vi "FP_pattern.vi"() -> ()   [LabVIEW 2014]
uses:
  Between.vi
panel:
  out "output cluster":cluster{i16, "Bottom":i16}
  in  "stop":bool caption="(F4)"
  in  "Picture":picture
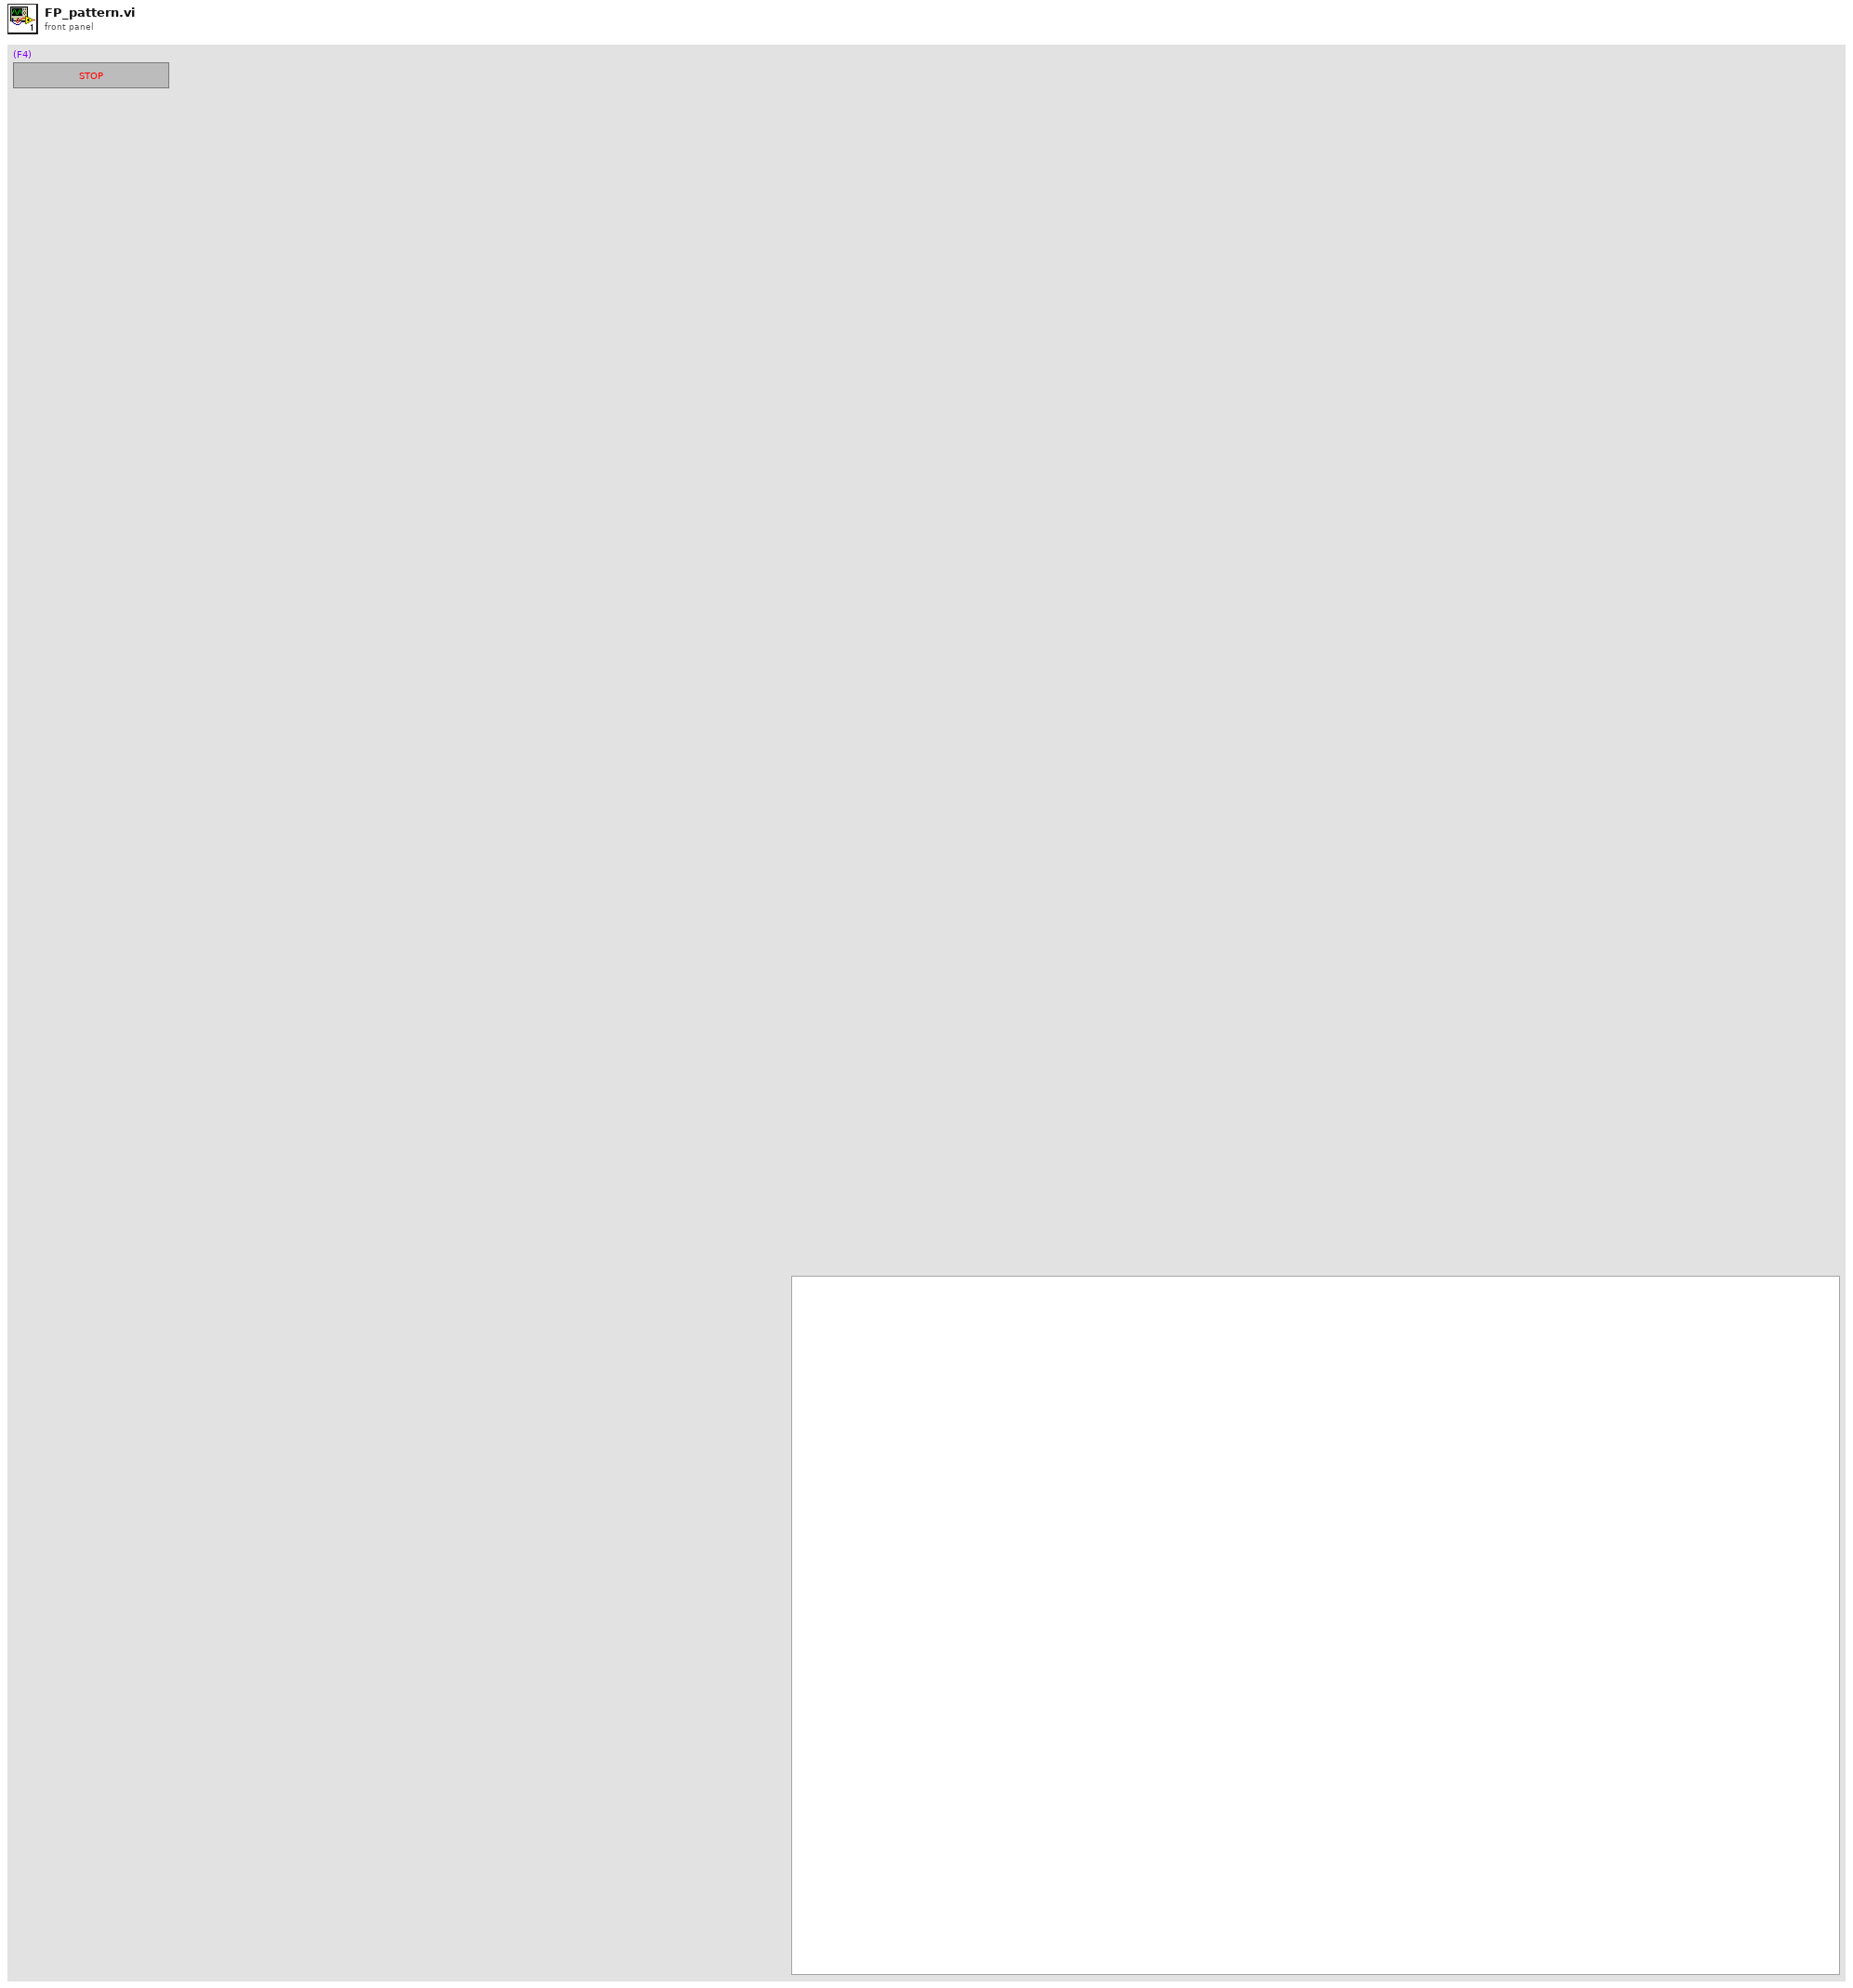
[diagram p1: front panel]
types:
  T1 = typedef "LVAllMonitorsDisplayTypeDef.ctl" = cluster{"Bounds":cluster{"Left":i16, "Top":i16, "Right":i16, "Bottom":i16}, "Depth":i16}[]
  T2 = cluster{"Bounds":cluster{"Left":i16, "Top":i16, "Right":i16, "Bottom":i16}, "Depth":i16}
  T3 = cluster{"Left":i16, "Top":i16, "Right":i16, "Bottom":i16}
  T4 = cluster{"Width":u16, "Style":enum32{"Solid", "Dash", "Dot", "DashDot", "DashDotDot"}}
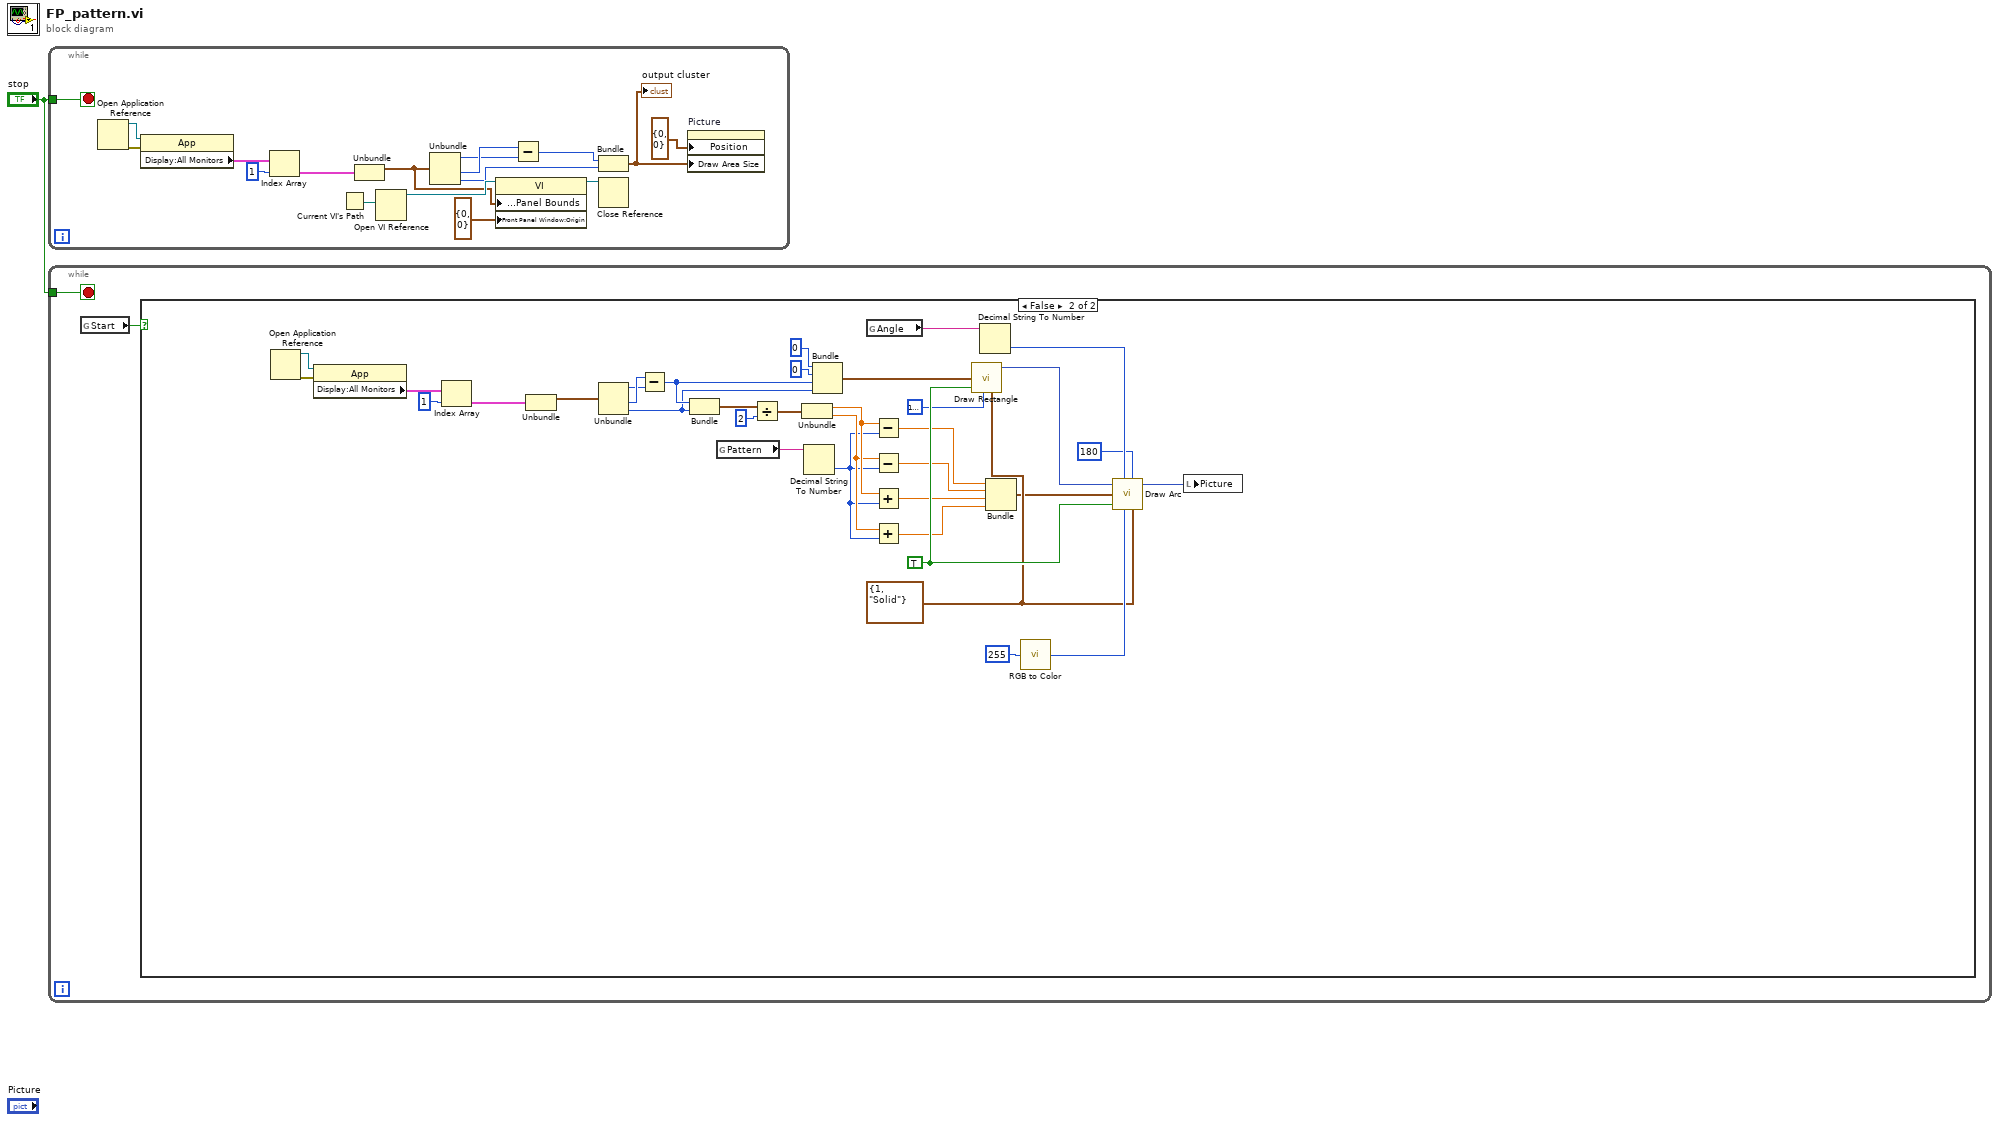
[diagram p0: block diagram]
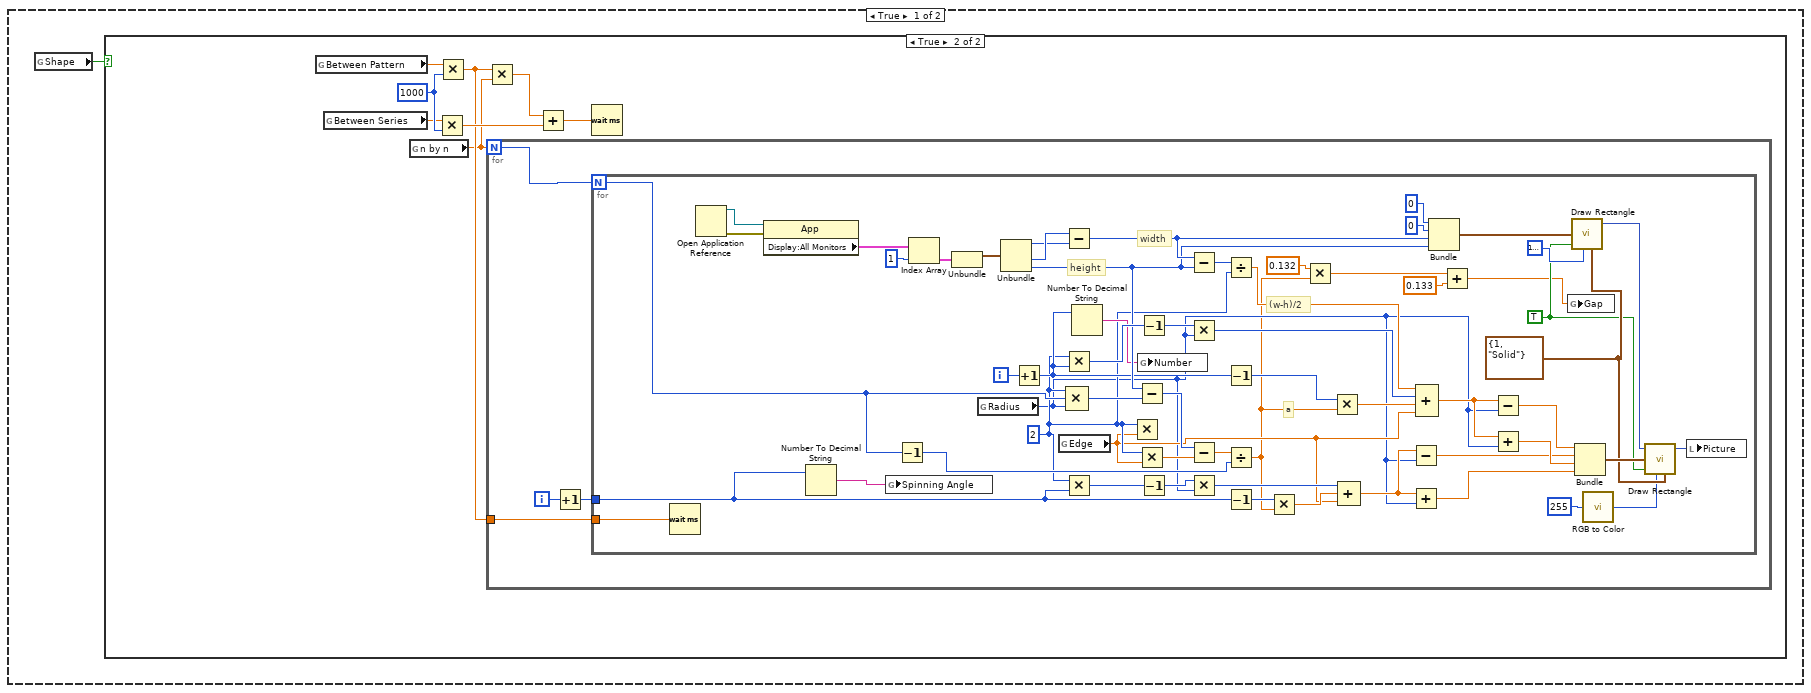
[diagram p2: hidden frame]
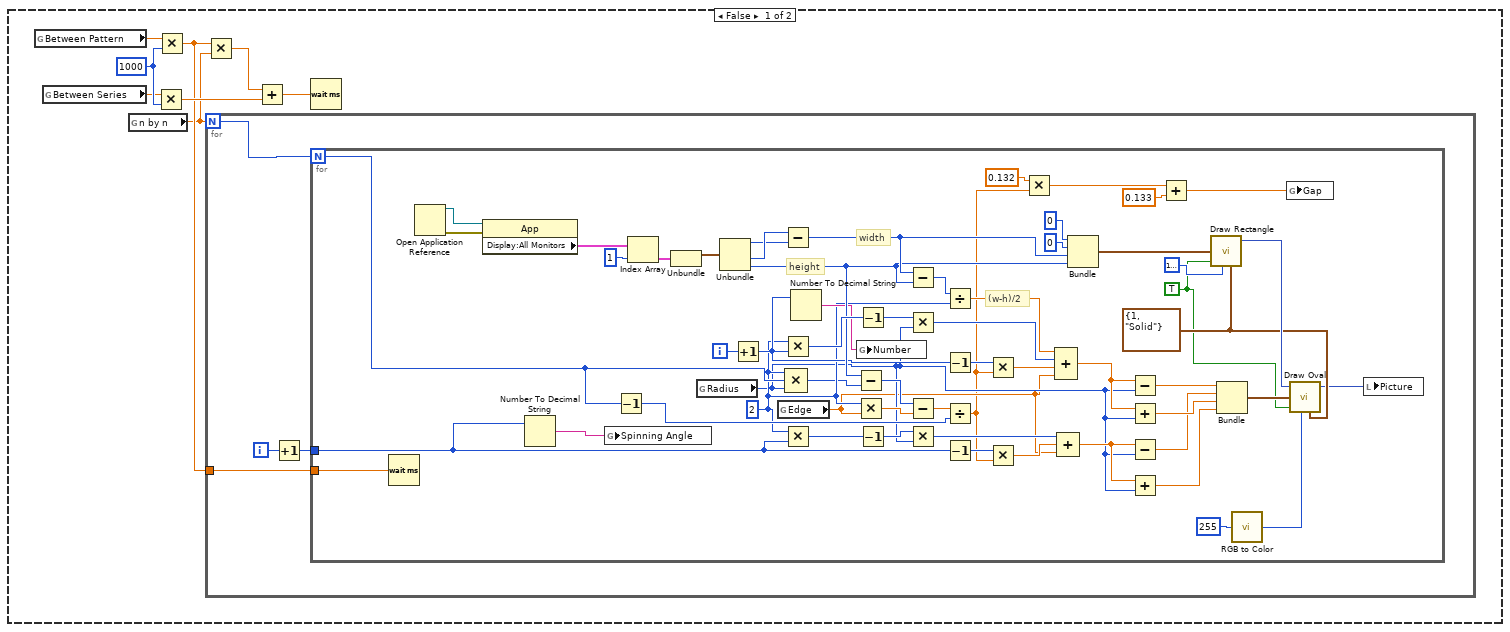
[diagram p3: hidden frame]
diagram:
  n1 = while {
    tunnel: "stop" -> [w13]
    stop <- w13 stop-if-true
    n2 = Open Application Reference() -> (0:w11:errorcluster, 3:w12:refnum<vi>)  [unwired: 1 in, 3 out]
    n3 = property class="App"(reference=w12, error in=w11) -> ("Display:All Monitors"=w10:T1)  [unwired: 2 out]
    n4 = Index Array(array=w10, index=1) -> (element=w8:T2)
    n5 = Current VI's Path() -> (path=w16:path)
    n6 = Unbundle(w8) -> ("Bounds"=w3:T3)  [unwired: 1 out]
    n7 = Open VI Reference(vi path=w16) -> (vi reference=w17:refnum<vi>)  [unwired: 5 in, 1 out]
    n8 = Unbundle(w3) -> ("Left"=w6:i16, "Right"=w7:i16, "Bottom"=w4:i16)  [unwired: 1 out]
    n9 = property class="VI"(reference=w17, "Front Panel Window:Panel Bounds"=w3, "Front Panel Window:Origin"=cluster{"Horizontal":i16, "Vertical":i16} {"Horizontal"=0, "Vertical"=0}) -> (reference out=w18:refnum<vi>)  [unwired: 1 in, 1 out]
    n10 = Subtract(x=w7, y=w6) -> (x-y=w5:i16)
    n11 = Bundle(w5, "Bottom"=w4) -> (w2:cluster{i16, "Bottom":i16})  [unwired: 1 in]
    "output cluster" <- w2
    n12 = Close Reference(reference=w18) -> ()  [unwired: 1 in, 1 out]
    n13 = property on="Picture" class="Pict"("Position"=cluster{"Left":i32, "Top":i32} {"Left"=0, "Top"=0}, "Draw Area Size"=w2) -> ()  [unwired: 2 in, 2 out]
  }
  n14 = while {
    tunnel: "stop" -> [w20]
    stop <- w20 stop-if-true
    n15 = global read "Between.vi" "Start"() -> (w19:bool)
    n16 = case shown="False" w19 {
      frame True {
        n17 = global read "Between.vi" "Shape"() -> (w21:bool)
        n18 = case shown="True" w21 {
          frame False {
            w26 = 1000
            n19 = global read "Between.vi" "Between Pattern"() -> (w23:dbl)
            n20 = global read "Between.vi" "Between Series"() -> (w24:dbl)
            n21 = global read "Between.vi" "n by n"() -> (w22:dbl)
            n22 = Multiply(x=w24, y=w26) -> (x*y=w27:dbl)
            n23 = Multiply(x=w23, y=w26) -> (x*y=w25:dbl)
            n24 = Multiply(x=w25, y=w22) -> (x*y=w29:dbl)
            n25 = for {
              N: w22 -> [w32]
              tunnel: w25 -> [w33]
              i -> [w31]
              n26 = Increment(x=w31) -> (x+1=w30:i32)
              n27 = for {
                N: w32 -> [w70]
                tunnel: w33 -> [w92]
                tunnel: w30 -> [w48]
                i -> [w59]
                w42 = 2
                w77 = T4 {"Width"=1, "Style"=enum."Solid"} ("pen")
                w75 = TRUE
                # "(w-h)/2"
                # "height"
                # "width"
                n28 = Wait (ms)(milliseconds to wait=w92) -> ()  [unwired: 1 out]
                n29 = Open Application Reference() -> (0:w90:errorcluster, 3:w91:refnum<vi>)  [unwired: 1 in, 3 out]
                n30 = property class="App"(reference=w91, error in=w90) -> ("Display:All Monitors"=w89:T1)  [unwired: 2 out]
                n31 = Number To Decimal String(number=w48) -> (decimal integer string=w47:string)  [unwired: 1 in]
                n32 = global write "Between.vi" "Spinning Angle"(w47) -> ()
                n33 = Decrement(x=w70) -> (x-1=w61:i32)
                n34 = Index Array(array=w89, index=1) -> (element=w88:T2)
                n35 = Unbundle(w88) -> ("Bounds"=w85:T3)  [unwired: 1 out]
                n36 = global read "Between.vi" "Radius"() -> (w41:i32)
                n37 = Unbundle(w85) -> ("Left"=w86:i16, "Right"=w87:i16, "Bottom"=w62:i16)  [unwired: 1 out]
                n38 = Increment(x=w59) -> (x+1=w45:i32)
                n39 = global read "Between.vi" "Edge"() -> (w40:dbl)
                n40 = Subtract(x=w87, y=w86) -> (x-y=w69:i16)
                n41 = Multiply(x=w42, y=w45) -> (x*y=w66:i32)
                n42 = Multiply(x=w42, y=w48) -> (x*y=w58:i32)
                n43 = Compound Arithmetic op=MULTIPLY(w42, w70, w41) -> (w34:i32)
                n44 = Number To Decimal String(number=w45) -> (decimal integer string=w46:string)  [unwired: 1 in]
                n45 = Subtract(x=w62, y=w34) -> (x-y=w71:i32)
                n46 = Multiply(x=w42, y=w40) -> (x*y=w43:dbl)
                n47 = global write "Between.vi" "Number"(w46) -> ()
                n48 = Decrement(x=w66) -> (x-1=w50:i32)
                n49 = Decrement(x=w58) -> (x-1=w52:i32)
                n50 = Subtract(x=w69, y=w62) -> (x-y=w68:i16)
                n51 = Multiply(x=w50, y=w41) -> (x*y=w49:i32)
                n52 = Subtract(x=w71, y=w43) -> (x-y=w53:dbl)
                n53 = Multiply(x=w52, y=w41) -> (x*y=w51:i32)
                n54 = Divide(x=w68, y=w42) -> (x/y=w67:dbl)
                n55 = Decrement(x=w45) -> (x-1=w65:i32)
                n56 = Divide(x=w53, y=w61) -> (x/y=w37:dbl)
                n57 = Decrement(x=w48) -> (x-1=w60:i32)
                n58 = Multiply(x=w65, y=w37) -> (x*y=w64:dbl)
                n59 = Multiply(x=w60, y=w37) -> (x*y=w57:dbl)
                n60 = Multiply(x=0.132, y=w37) -> (x*y=w39:dbl)
                n61 = Compound Arithmetic op=ADD(w67, w49, w64, w40) -> (w63:dbl)
                n62 = Compound Arithmetic op=ADD(w51, w57, w40) -> (w54:dbl)
                n63 = Bundle(0, 0, w69, "Bottom"=w62) -> (w84:cluster{i32, i32, i16, "Bottom":i16})  [unwired: 1 in]
                n64 = Subtract(x=w63, y=w41) -> (x-y=w79:dbl)
                n65 = Add(x=w63, y=w41) -> (x+y=w80:dbl)
                n66 = Subtract(x=w54, y=w41) -> (x-y=w55:dbl)
                n67 = Add(x=w54, y=w41) -> (x+y=w56:dbl)
                n68 = Add(x=w39, y=0.133) -> (x+y=w35:dbl)
                n69 = call <vilib>:"Draw Rectangle.vi"("rect"=w84, "fill?(F)"=w75, "color(black)"=u32 16777222, "pen"=w77) -> ("new picture"=w78:picture)  [unwired: 5 in]
                n70 = Bundle(w79, w55, w80, w56) -> (w81:cluster{dbl, dbl, dbl, dbl})  [unwired: 1 in]
                n71 = call <vilib>:"RGB to Color.vi"("G"=255) -> ("Color"=w73:u32)  [unwired: 2 in]
                n72 = global write "Between.vi" "Gap"(w35) -> ()
                n73 = call <vilib>:"Draw Oval.vi"("picture"=w78, "rect"=w81, "fill?(F)"=w75, "color(black)"=w73, "pen"=w77) -> ("new picture"=w44:picture)  [unwired: 4 in]
                n74 = local write "Picture"(w44) -> ()
              }
            }
            n75 = Add(x=w29, y=w27) -> (x+y=w28:dbl)
            n76 = Wait (ms)(milliseconds to wait=w28) -> ()  [unwired: 1 out]
          }
          frame True {
            w97 = 1000
            n77 = global read "Between.vi" "Between Pattern"() -> (w94:dbl)
            n78 = global read "Between.vi" "Between Series"() -> (w95:dbl)
            n79 = global read "Between.vi" "n by n"() -> (w93:dbl)
            n80 = Multiply(x=w95, y=w97) -> (x*y=w98:dbl)
            n81 = Multiply(x=w94, y=w97) -> (x*y=w96:dbl)
            n82 = Multiply(x=w96, y=w93) -> (x*y=w100:dbl)
            n83 = for {
              N: w93 -> [w103]
              tunnel: w96 -> [w104]
              i -> [w102]
              n84 = Increment(x=w102) -> (x+1=w101:i32)
              n85 = for {
                N: w103 -> [w140]
                tunnel: w104 -> [w163]
                tunnel: w101 -> [w118]
                i -> [w129]
                w112 = 2
                w148 = T4 {"Width"=1, "Style"=enum."Solid"} ("pen")
                w146 = TRUE
                # "a"
                # "(w-h)/2"
                # "height"
                # "width"
                n86 = Wait (ms)(milliseconds to wait=w163) -> ()  [unwired: 1 out]
                n87 = Open Application Reference() -> (0:w161:errorcluster, 3:w162:refnum<vi>)  [unwired: 1 in, 3 out]
                n88 = property class="App"(reference=w162, error in=w161) -> ("Display:All Monitors"=w160:T1)  [unwired: 2 out]
                n89 = Number To Decimal String(number=w118) -> (decimal integer string=w117:string)  [unwired: 1 in]
                n90 = global write "Between.vi" "Spinning Angle"(w117) -> ()
                n91 = Decrement(x=w140) -> (x-1=w131:i32)
                n92 = Index Array(array=w160, index=1) -> (element=w159:T2)
                n93 = Unbundle(w159) -> ("Bounds"=w156:T3)  [unwired: 1 out]
                n94 = global read "Between.vi" "Radius"() -> (w110:i32)
                n95 = Unbundle(w156) -> ("Left"=w157:i16, "Right"=w158:i16, "Bottom"=w132:i16)  [unwired: 1 out]
                n96 = Increment(x=w129) -> (x+1=w115:i32)
                n97 = global read "Between.vi" "Edge"() -> (w111:dbl)
                n98 = Subtract(x=w158, y=w157) -> (x-y=w139:i16)
                n99 = Multiply(x=w112, y=w115) -> (x*y=w136:i32)
                n100 = Multiply(x=w112, y=w118) -> (x*y=w128:i32)
                n101 = Compound Arithmetic op=MULTIPLY(w112, w140, w110) -> (w142:i32)
                n102 = Number To Decimal String(number=w115) -> (decimal integer string=w116:string)  [unwired: 1 in]
                n103 = Multiply(x=w112, y=w111) -> ()  [unwired: 1 out]
                n104 = Subtract(x=w132, y=w142) -> (x-y=w141:i32)
                n105 = Multiply(x=w112, y=w111) -> (x*y=w113:dbl)
                n106 = global write "Between.vi" "Number"(w116) -> ()
                n107 = Decrement(x=w136) -> (x-1=w120:i32)
                n108 = Decrement(x=w128) -> (x-1=w122:i32)
                n109 = Subtract(x=w139, y=w132) -> (x-y=w138:i16)
                n110 = Multiply(x=w120, y=w110) -> (x*y=w119:i32)
                n111 = Subtract(x=w141, y=w113) -> (x-y=w123:dbl)
                n112 = Multiply(x=w122, y=w110) -> (x*y=w121:i32)
                n113 = Divide(x=w138, y=w112) -> (x/y=w137:dbl)
                n114 = Decrement(x=w115) -> (x-1=w135:i32)
                n115 = Divide(x=w123, y=w131) -> (x/y=w107:dbl)
                n116 = Decrement(x=w118) -> (x-1=w130:i32)
                n117 = Multiply(x=w130, y=w107) -> (x*y=w127:dbl)
                n118 = Multiply(x=0.132, y=w107) -> (x*y=w109:dbl)
                n119 = Multiply(x=w135, y=w107) -> (x*y=w134:dbl)
                n120 = Compound Arithmetic op=ADD(w121, w127, w111) -> (w124:dbl)
                n121 = Subtract(x=w124, y=w110) -> (x-y=w125:dbl)
                n122 = Add(x=w124, y=w110) -> (x+y=w126:dbl)
                n123 = Compound Arithmetic op=ADD(w137, w119, w134, w111) -> (w133:dbl)
                n124 = Bundle(0, 0, w139, "Bottom"=w132) -> (w155:cluster{i32, i32, i16, "Bottom":i16})  [unwired: 1 in]
                n125 = Add(x=w109, y=0.133) -> (x+y=w105:dbl)
                n126 = Subtract(x=w133, y=w110) -> (x-y=w150:dbl)
                n127 = Add(x=w133, y=w110) -> (x+y=w151:dbl)
                n128 = global write "Between.vi" "Gap"(w105) -> ()
                n129 = call <vilib>:"Draw Rectangle.vi"("rect"=w155, "fill?(F)"=w146, "color(black)"=u32 16777222, "pen"=w148) -> ("new picture"=w149:picture)  [unwired: 5 in]
                n130 = Bundle(w150, w125, w151, w126) -> (w152:cluster{dbl, dbl, dbl, dbl})  [unwired: 1 in]
                n131 = call <vilib>:"RGB to Color.vi"("G"=255) -> ("Color"=w144:u32)  [unwired: 2 in]
                n132 = call <vilib>:"Draw Rectangle.vi"("picture"=w149, "rect"=w152, "fill?(F)"=w146, "color(black)"=w144, "pen"=w148) -> ("new picture"=w114:picture)  [unwired: 4 in]
                n133 = local write "Picture"(w114) -> ()
              }
            }
            n134 = Add(x=w100, y=w98) -> (x+y=w99:dbl)
            n135 = Wait (ms)(milliseconds to wait=w99) -> ()  [unwired: 1 out]
          }
        }
      }
      frame False {
        w194 = T4 {"Width"=1, "Style"=enum."Solid"} ("pen")
        w196 = TRUE
        n136 = Open Application Reference() -> (0:w180:errorcluster, 3:w181:refnum<vi>)  [unwired: 1 in, 3 out]
        n137 = property class="App"(reference=w181, error in=w180) -> ("Display:All Monitors"=w179:T1)  [unwired: 2 out]
        n138 = Index Array(array=w179, index=1) -> (element=w177:T2)
        n139 = Unbundle(w177) -> ("Bounds"=w174:T3)  [unwired: 1 out]
        n140 = Unbundle(w174) -> ("Left"=w175:i16, "Right"=w176:i16, "Bottom"=w171:i16)  [unwired: 1 out]
        n141 = Subtract(x=w176, y=w175) -> (x-y=w172:i16)
        n142 = Bundle(w172, "Bottom"=w171) -> (w173:cluster{i16, "Bottom":i16})  [unwired: 1 in]
        n143 = global read "Between.vi" "Pattern"() -> (w165:string)
        n144 = Divide(x=w173, y=2) -> (x/y=w185:cluster{dbl, "Bottom":dbl})
        n145 = Unbundle(w185) -> (w183:dbl, "Bottom"=w182:dbl)
        n146 = Decimal String To Number(string=w165) -> (number=w164:i32)  [unwired: 2 in, 1 out]
        n147 = Bundle(0, 0, w172, "Bottom"=w171) -> (w184:cluster{i32, i32, i16, "Bottom":i16})  [unwired: 1 in]
        n148 = global read "Between.vi" "Angle"() -> (w170:string)
        n149 = Subtract(x=w183, y=w164) -> (x-y=w190:dbl)
        n150 = Subtract(x=w182, y=w164) -> (x-y=w192:dbl)
        n151 = Add(x=w183, y=w164) -> (x+y=w189:dbl)
        n152 = Add(x=w182, y=w164) -> (x+y=w191:dbl)
        n153 = call <vilib>:"Draw Rectangle.vi"("rect"=w184, "fill?(F)"=w196, "color(black)"=u32 16777222, "pen"=w194) -> ("new picture"=w193:picture)  [unwired: 5 in]
        n154 = Decimal String To Number(string=w170) -> (number=w169:i32)  [unwired: 2 in, 1 out]
        n155 = Bundle(w190, w192, w189, w191) -> (w166:cluster{dbl, dbl, dbl, dbl})  [unwired: 1 in]
        n156 = call <vilib>:"RGB to Color.vi"("G"=255) -> ("Color"=w198:u32)  [unwired: 2 in]
        n157 = call <vilib>:"Draw Arc.vi"("picture"=w193, "start angle[degrees]"=w169, "rect"=w166, "fill?(F)"=w196, "color(black)"=w198, "arc size[degrees]"=180, "pen"=w194) -> ("new picture"=w167:picture)  [unwired: 2 in]
        n158 = local write "Picture"(w167) -> ()
      }
    }
  }
